vi "Run Service.vi"() -> ()   [LabVIEW 2020, in "NI-DMM Measurement.lvlib"]
uses:
  NI-DMM Measurement.lvlib
  RPC Service/MeasurementService/MeasurementService.lvclass
  C:/Program Files/National Instruments/LabVIEW 2020/vi.lib/gRPC/LabVIEW gRPC Servicer/ServiceBase/ServiceBase.lvclass
  <vilib>/gRPC/LabVIEW gRPC Servicer/Servicer/Servicer.lvclass/Servicer.ctl
  <vilib>/gRPC/LabVIEW gRPC Servicer/Servicer/Servicer.lvclass
  <vilib>/MeasurementLink/MeasurementLink Measurement Server Internal/MeasurementLink Measurement Server Internal.lvlib
  <vilib>/MeasurementLink/Discovery Client/MeasurementLink Discovery Client.lvlib
panel:
  out "Listening Port":i32
  in  "Stop":bool
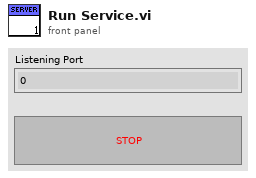
[diagram p1: front panel]
types:
  T1 = enum32{"Invalid", "Standard", "Closed", "Hidden", "Minimized", "Maximized"}
  T2 = typedef "grpc-lvsupport-release.lvlib/grpcId.ctl" = u64
  T3 = typedef "MeasurementLink Discovery Client.lvlib/ni_measurementlink_discovery_v1_RegisterServiceResponse.ctl" = cluster{"registration_id":string}
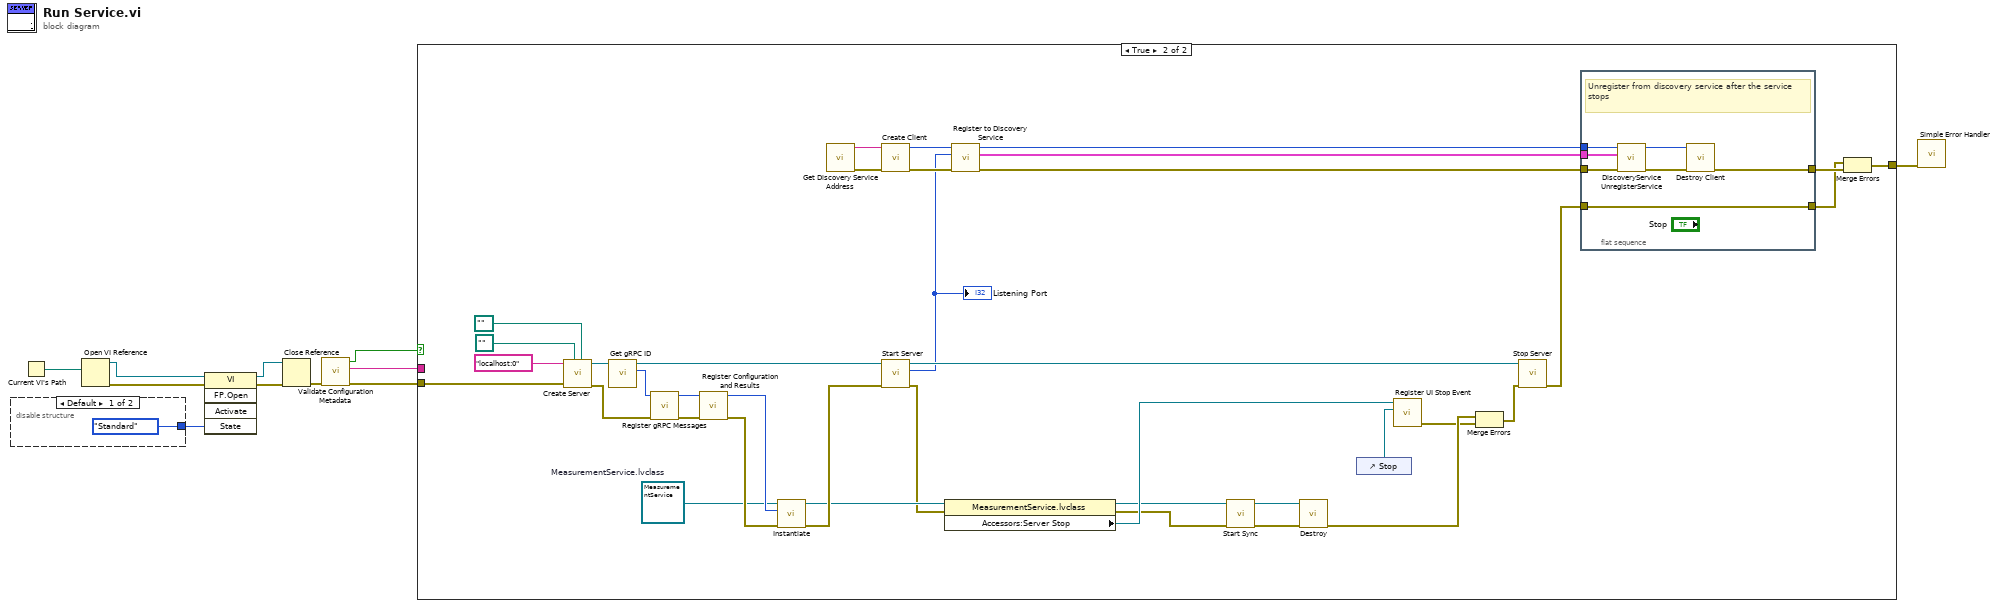
[diagram p0: block diagram]
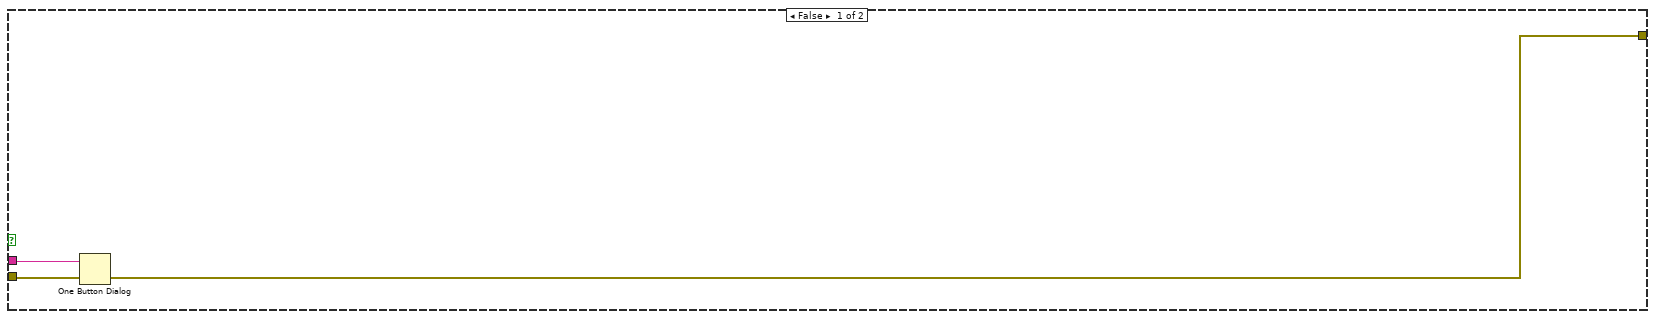
[diagram p2: hidden frame]
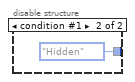
[diagram p3: hidden frame]
diagram:
  n1 = disable-structure shown="Default" {
    disable-tunnel: [T1."Standard" ("State") T1."Hidden" ("State")] -> w6
    frame condition #0 (active) {
    }
    frame condition #1 {
    }
  }
  n2 = Current VI's Path() -> (path=w10:path)
  n3 = Open VI Reference(vi path=w10) -> (vi reference=w7:refnum<vi>, error out=w9:errorcluster)  [unwired: 5 in]
  n4 = invoke class="VI" method="FP.Open"(reference=w7, error in=w9, "State"=w6) -> (reference out=w5:refnum<vi>, error out=w8:errorcluster)  [unwired: 2 in, 3 out]
  n5 = Close Reference(reference=w5, error in (no error)=w8) -> (error out=w4:errorcluster)
  n6 = call "Validate Configuration Metadata.vi"("error in (no error)"=w4) -> ("error out"=w3:errorcluster, "Invalid Parameters"=w1:string, "Is Metadata Valid"=w2:bool)  [unwired: 8 in]
  n7 = case shown="True" w2 {
    tunnel: [w14 w35] -> w11
    tunnel: w3 -> [w14 w17]
    tunnel: w1 -> [w15 _]
    frame False {
      n8 = One Button Dialog(message=w15) -> ()  [unwired: 1 in, 1 out]
    }
    frame True {
      w16 = refnum<class "MeasurementService.lvclass"> refnum  # MeasurementService.lvclass
      n9 = call <vilib>:"Create Server.vi"("Server Key File (.key)"=path "", "Server Certificate File (.crt)"=path "", "error in"=w17, "Server Address"="localhost:0") -> ("error out"=w47:errorcluster, "gRPC Server out"=w49:refnum<class "Servicer.lvclass">)  [unwired: 6 in]
      n10 = call <vilib>:"Get gRPC ID.vi"("OOP Server in"=w49) -> ("gRPC ID"=w48:T2, "OOP Server out"=w44:refnum<class "Servicer.lvclass">)  [unwired: 9 in]
      n11 = call <vilib>:"Register gRPC Messages.vi"("error in (no error)"=w47, "gRPC ID"=w48) -> ("error out"=w31:errorcluster, "gRPC ID Out"=w32:T2)  [unwired: 8 in]
      n12 = call "Register Configuration and Results.vi"("error in (no error)"=w31, "gRPC ID"=w32) -> ("error out"=w30:errorcluster, "gRPC ID Out"=w28:T2)  [unwired: 8 in]
      n13 = call-dynamic "Instantiate.vi"("error in"=w30, "gRPCid"=w28, "iService"=w16) -> ("error out"=w24:errorcluster, "iService"=w23:refnum<class "MeasurementService.lvclass">)  [unwired: 7 in]
      n14 = call "Get Discovery Service Address.vi"() -> ("error out"=w19:errorcluster, "address"=w18:string)  [unwired: 10 in]
      n15 = call <vilib>:"Create Client.vi"("error in"=w19, "address"=w18) -> ("error out"=w41:errorcluster, "gRPC ID Out"=w42:T2)  [unwired: 8 in]
      n16 = call <vilib>:"Start Server.vi"("error in"=w24, "gRPC Server in"=w44) -> ("error out"=w22:errorcluster, "Listening Port"=w29:i32, "gRPC Server out"=w53:refnum<class "Servicer.lvclass">)  [unwired: 7 in]
      "Listening Port" <- w29
      n17 = property class="MeasurementService.lvclass"(reference=w23, error in=w22) -> (reference out=w20:refnum<class "MeasurementService.lvclass">, error out=w21:errorcluster, "Accessors:Server Stop"=w25:refnum<user-event>)
      n18 = call "Register to Discovery Service.vi"("error in"=w41, "PortNumber"=w29, "gRPC ID"=w42) -> ("error out"=w39:errorcluster, "Response Data"=w38:T3, "gRPC ID out"=w40:T2)  [unwired: 6 in]
      n19 = call-dynamic "Start Sync.vi"("error in (no error)"=w21, "gRPC Server in"=w20) -> ("error out"=w46:errorcluster, "gRPC Server out"=w45:refnum<class "MeasurementService.lvclass">)  [unwired: 8 in]
      n20 = call-dynamic "Destroy.vi"("error in (no error)"=w46, "SignalGeneratorService in"=w45) -> ("error out"=w27:errorcluster)  [unwired: 8 in, 1 out]
      n21 = control-ref of="Stop"() -> (w37:refnum<vi>)
      n22 = call "Register UI Stop Event.vi"("Stop Button [ref]"=w37, "Server Stop"=w25) -> ("error out"=w26:errorcluster)  [unwired: 9 in]
      n23 = Merge Errors(w27, w26) -> (w43:errorcluster)
      n24 = call <vilib>:"Stop Server.vi"("error in"=w43, "gRPC Server in"=w53) -> ("error out"=w33:errorcluster)  [unwired: 9 in]
      n25 = flat-sequence {
        tunnel: w40 -> [w60]
        tunnel: w39 -> [w59]
        tunnel: w38 -> [w58]
        tunnel: [w55] -> w36
        tunnel: [w54] -> w34
        tunnel: w33 -> [w54]
        frame #0 {
          # "Unregister from discovery service after the service stops"
          n26 = call <vilib>:"DiscoveryService UnregisterService.vi"("error in"=w59, "Request Data"=w58, "gRPC ID"=w60) -> ("error out"=w56:errorcluster, "gRPC ID out"=w57:T2)  [unwired: 6 in, 1 out]
          n27 = call <vilib>:"Destroy Client.vi"("error in"=w56, "gRPC ID"=w57) -> ("error out"=w55:errorcluster)  [unwired: 9 in]
        }
      }
      n28 = Merge Errors(w34, w36) -> (w35:errorcluster)
    }
  }
  n29 = call <vilib>:"Simple Error Handler.vi"("error in (no error)"=w11) -> ()  [unwired: 4 in, 5 out]
